vi "AG33XXX.ProcCases.vi"(0 "i ref in":refnum<vi>, 1 "selector":string, 2 "Data":T1, 3 "call cluster":T2={"Object"="", "Selector"="", "CallType"=enum."synchronous", "Async Object"="", "Async Selector"="", "Data Descriptor"="", "Data"=[], "Error #"=0, "Expire"=0}, 5 "error in (no error)":errorcluster) -> (14 "i ref out":refnum<vi>, 17 "answer cluster":T2={"Object"="", "Selector"="", "CallType"=enum."synchronous", "Async Object"="", "Async Selector"="", "Data Descriptor"="", "Data"=[], "Error #"=0, "Expire"=0}, 19 "error out":errorcluster)   [LabVIEW 2014, in "AG33XXX.lvlib"]
doc: "This method is called by a process from within the default case in the event loop. The methods of a class that are linked to events will be called from THIS method. Add your code here."
uses:
  AG33XXX.lvlib
  CSCore/CSSystem/CoreDefs/CoreDefs.call_type.ctl
  CSCore/BaseProcess/BaseProcess.descriptor string definition.ctl
  CSCore/CSSystem/CoreDefs/CoreDefs.rawDataType.ctl
  CSCore/CSSystem/CoreLib/CoreLib.string 2 byte array.vi
  CSCore/CSSystem/CoreLib/CoreLib.byte array 2 short.vi
  CSCore/CSSystem/CoreLib/CoreLib.byte array 2 string.vi
  CSCore/CSSystem/CoreLib/CoreLib.byte array 2 short array.vi
  CSCore/CSSystem/CoreLib/CoreLib.byte array 2 double.vi
  CSCore/CSSystem/CoreLib/CoreLib.lvlib
  CSCore/BaseProcess/BaseProcess.lvlib
  CSCore/CSApplicationBaseClasses/AFGBase/AFGBase.lvlib
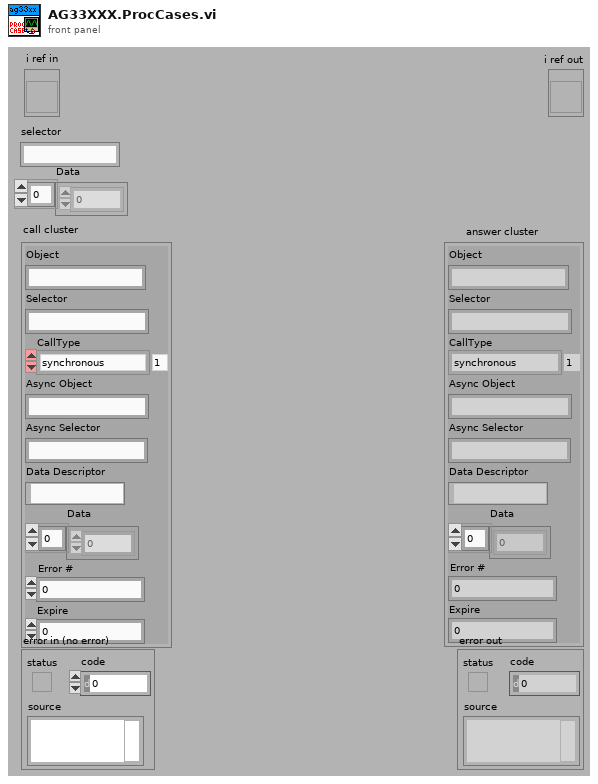
[diagram p1: front panel]
types:
  T1 = typedef "CoreDefs.rawDataType.ctl" = i8[]
  T2 = typedef "CoreDefs.call_type.ctl" = cluster{"Object":string, "Selector":string, "CallType":enum16{"simple", "synchronous", "asynchronous"}, "Async Object":string, "Async Selector":string, "Data Descriptor":T3, "Data":T1, "Error #":i32, "Expire":u32}
  T3 = typedef "BaseProcess.lvlib/BaseProcess.descriptor string definition.ctl" = string
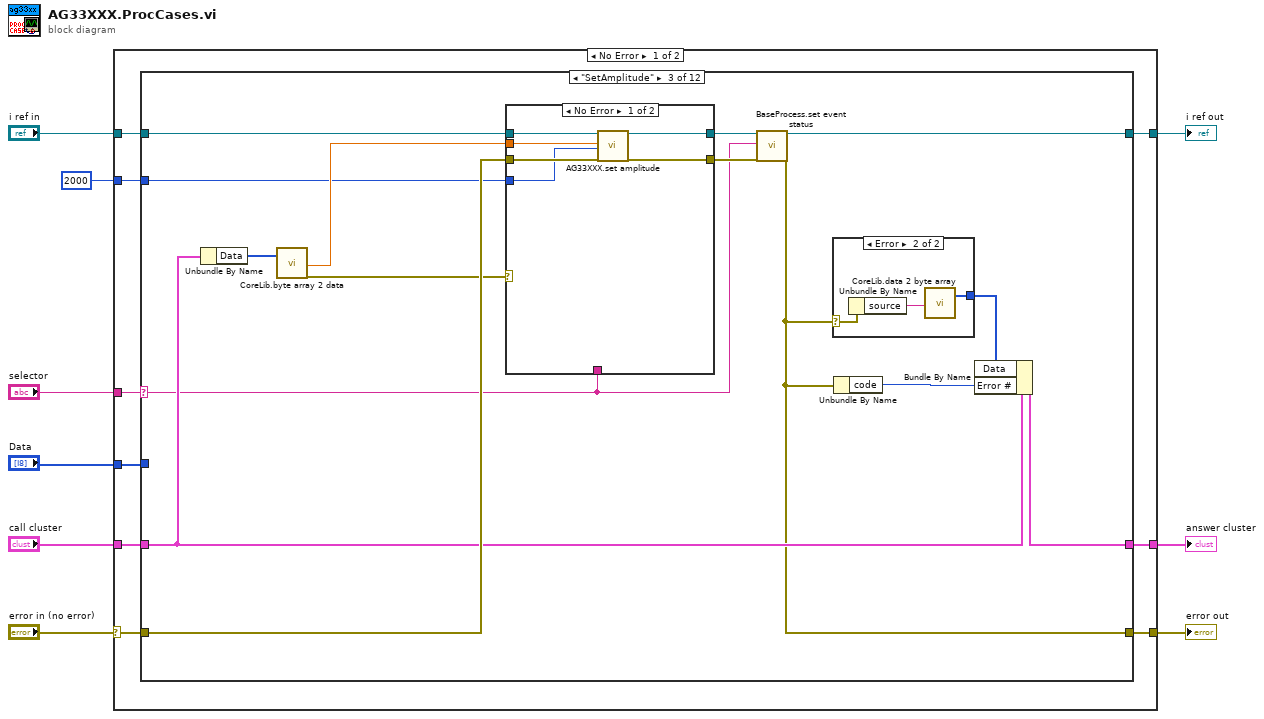
[diagram p0: block diagram]
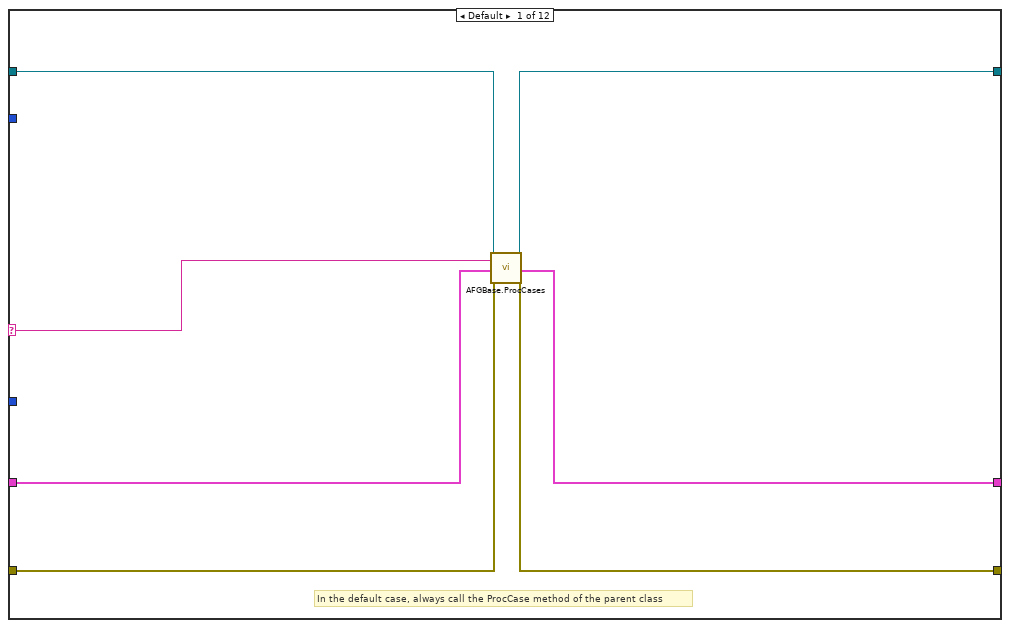
[diagram p2: hidden frame]
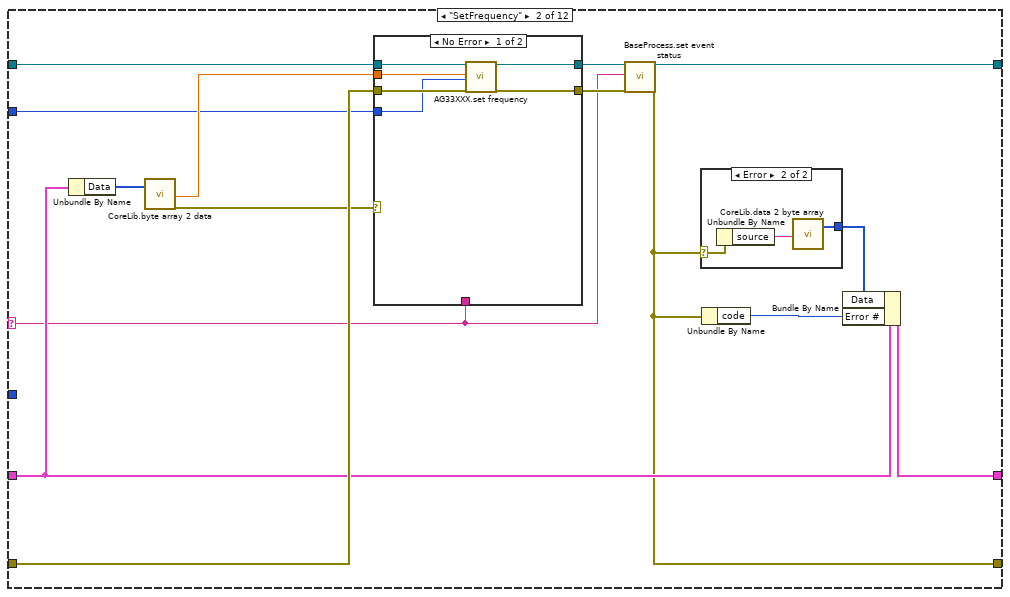
[diagram p3: hidden frame]
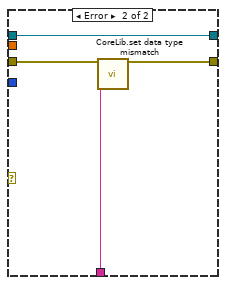
[diagram p5: hidden frame]
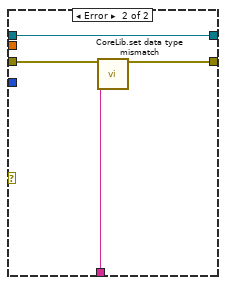
[diagram p7: hidden frame]
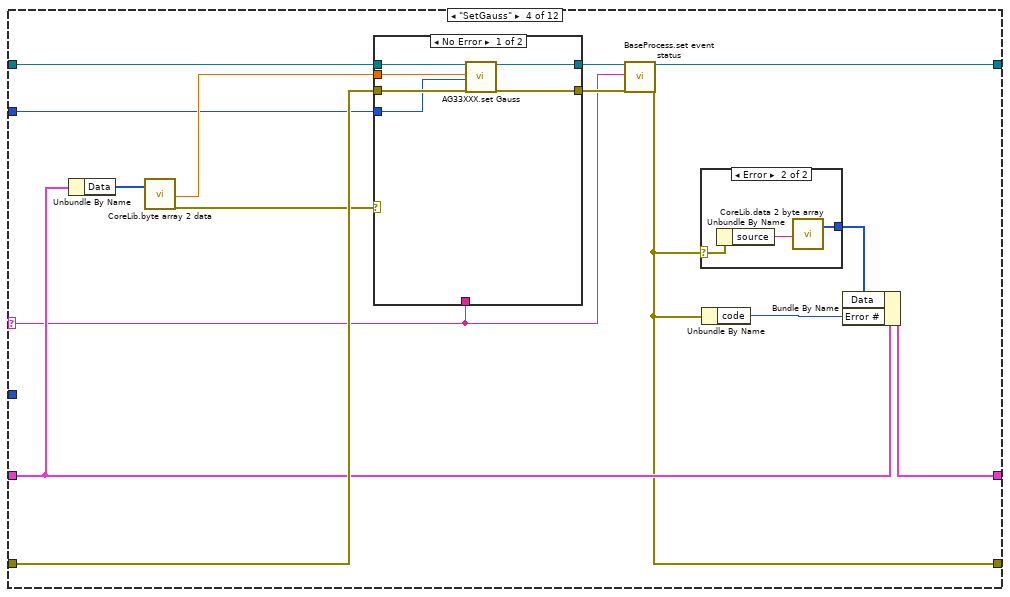
[diagram p8: hidden frame]
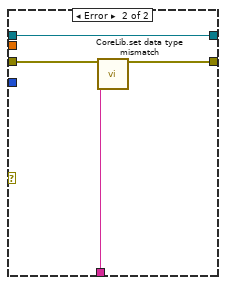
[diagram p10: hidden frame]
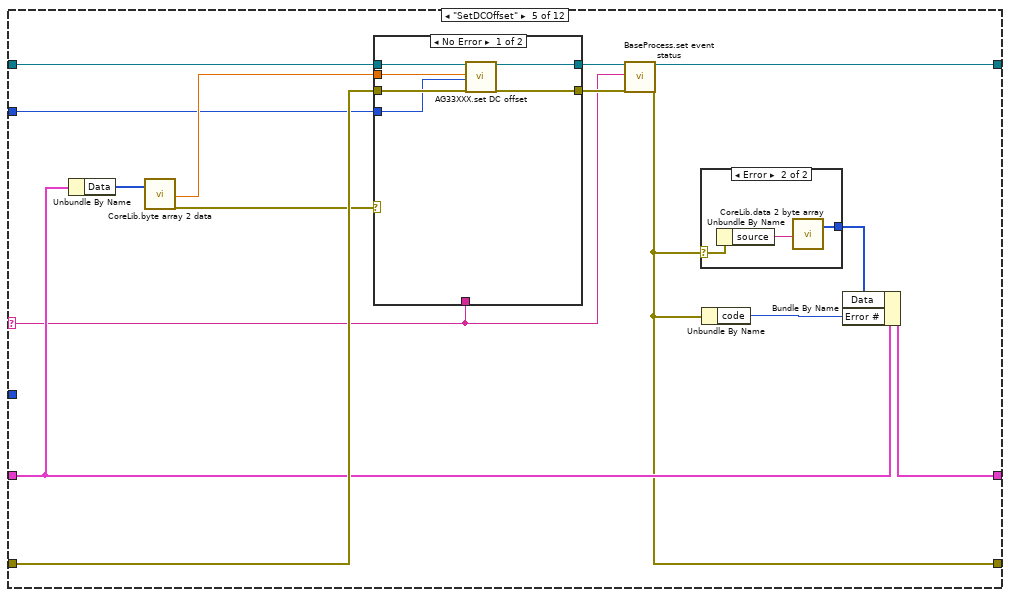
[diagram p11: hidden frame]
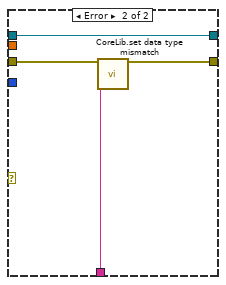
[diagram p13: hidden frame]
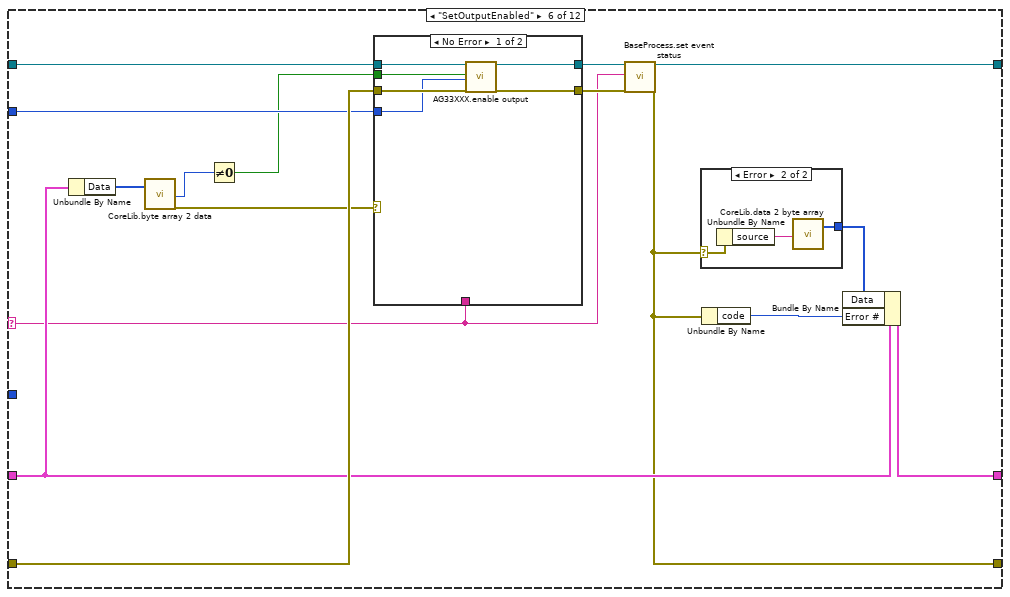
[diagram p14: hidden frame]
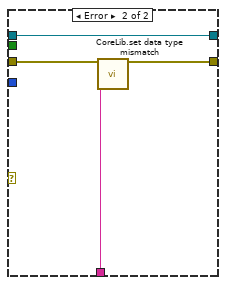
[diagram p16: hidden frame]
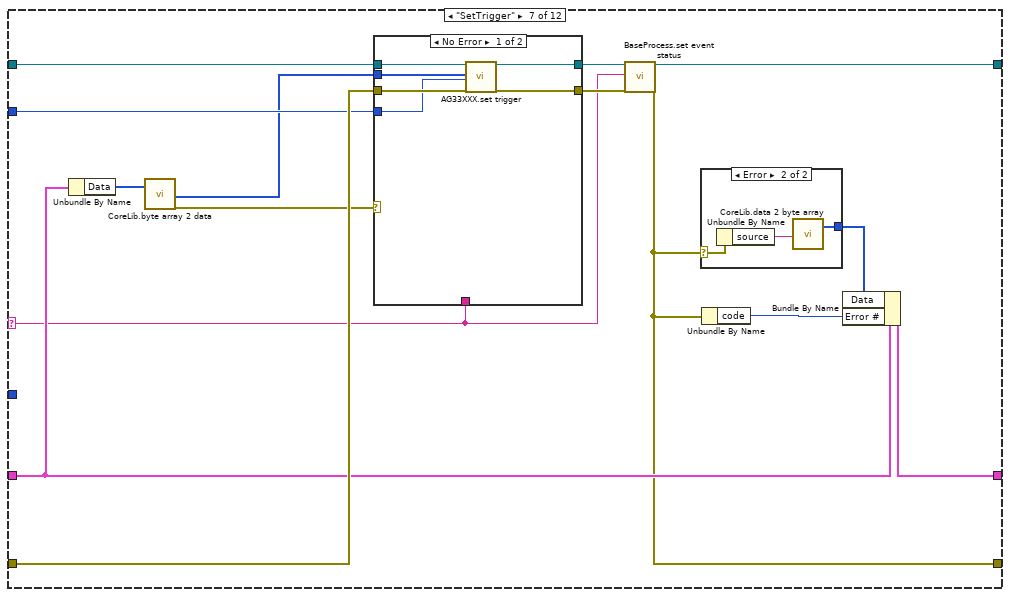
[diagram p17: hidden frame]
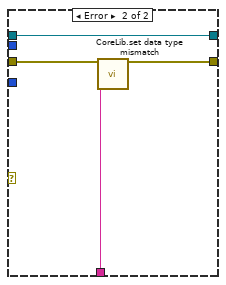
[diagram p19: hidden frame]
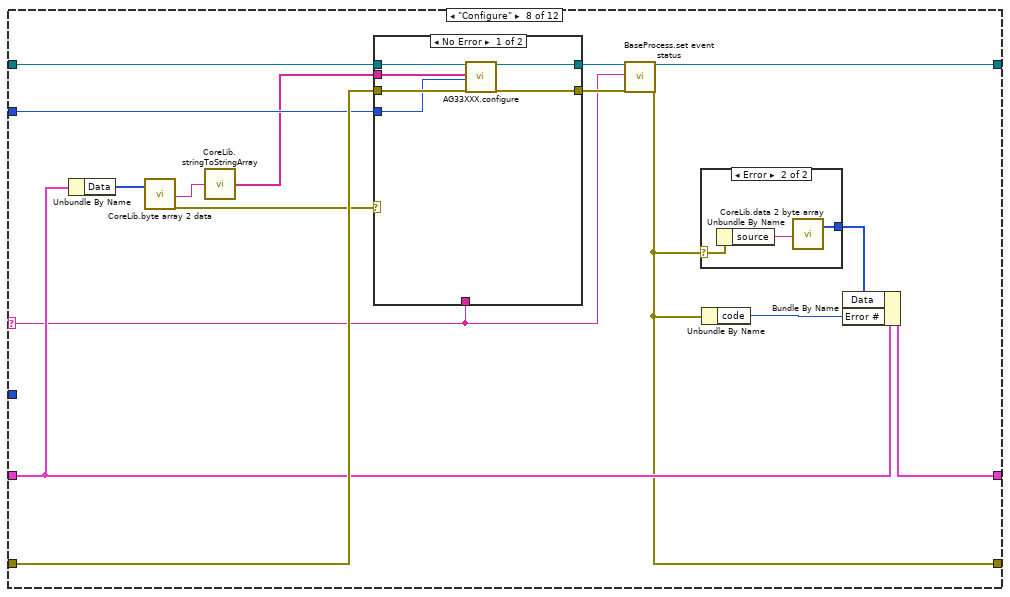
[diagram p20: hidden frame]
diagram:
  n1 = case shown="No Error" "error in (no error)" {
    selector: "error in (no error)" -> [w11 w310]
    tunnel: "selector" -> [w18 _]
    tunnel: [w17 w311] -> w8
    tunnel: "Data" -> [w16 _]
    tunnel: "call cluster" -> [w15 w311]
    tunnel: "i ref in" -> [w14 w312]
    tunnel: [w13 w312] -> w4
    tunnel: [w12 w310] -> w3
    tunnel: 2000 ("ms timeout (10000)") -> [w10 _]
    frame No Error {
      n2 = case shown="\"SetAmplitude\"" w18 {
        selector: w18 -> [w20 w31 w59 w87 w115 w144 w172 w201 w226 w241 w286 w301]
        tunnel: w16 -> [_ _ _ _ _ _ _ _ _ _ _ _]
        tunnel: w14 -> [w19 w40 w68 w96 w124 w153 w181 w210 w235 w249 w282 w297]
        tunnel: [w25 w30 w58 w86 w114 w143 w171 w200 w225 w252 w285 w300] -> w13
        tunnel: w15 -> [w21 w37 w65 w93 w121 w150 w178 w207 w232 w245 w290 w305]
        tunnel: [w22 w36 w64 w92 w120 w149 w177 w206 w231 w257 w289 w304] -> w17
        tunnel: w11 -> [w24 w39 w67 w95 w123 w152 w180 w209 w234 w250 w283 w298]
        tunnel: [w23 w32 w60 w88 w116 w145 w173 w202 w227 w253 w287 w302] -> w12
        tunnel: w10 -> [_ w26 w54 w82 w110 w139 w168 w197 w224 w251 w284 w299]
        frame Default {
          # "In the default case, always call the ProcCase method of the parent class"
          n3 = call "AFGBase.ProcCases.vi"("i ref in"=w19, "selector"=w20, "call cluster"=w21, "error in (no error)"=w24) -> ("i ref out"=w25:refnum<vi>, "answer cluster"=w22:T2, "error out"=w23:errorcluster)  [unwired: 13 in]
        }
        frame "SetFrequency" {
          n4 = Unbundle By Name(w37) -> ("Data"=w29:T1)
          n5 = call-poly "CoreLib.byte array 2 data.vi"("byteArray"=w29) -> ("d64"=w28:dbl, "error out"=w27:errorcluster)  [unwired: 16 in, 1 out]
          n6 = case shown="No Error" w27 {
            tunnel: [w48 w53] -> w34
            tunnel: w40 -> [w49 w53]
            tunnel: w39 -> [w46 w52]
            tunnel: [w47 w51] -> w33
            tunnel: w31 -> [_ w50]
            tunnel: w28 -> [w45 _]
            tunnel: w26 -> [w44 _]
            frame No Error {
              n7 = call "AG33XXX.set frequency.vi"("i ref in"=w49, "frequency [Hz]"=w45, "ms timeout (10000)"=w44, "error in (no error)"=w46) -> ("i ref out"=w48:refnum<vi>, "error out"=w47:errorcluster)  [unwired: 13 in, 1 out]
            }
            frame Error {
              n8 = call "CoreLib.set data type mismatch.vi"("error in (no error)"=w52, "error source"=w50) -> ("error out"=w51:errorcluster)  [unwired: 17 in]
            }
          }
          n9 = call "BaseProcess.set event status.vi"("i ref in"=w34, "EventStatus"=w31, "error in (no error)"=w33) -> ("i ref out"=w30:refnum<vi>, "error out"=w32:errorcluster)  [unwired: 14 in, 1 out]
          n10 = case shown="Error" w32 {
            selector: w32 -> [_ w43]
            tunnel: [_ w42] -> w35
            frame No Error {
            }
            frame Error {
              n11 = Unbundle By Name(w43) -> ("source"=w41:string)
              n12 = call-poly "CoreLib.data 2 byte array.vi"("string"=w41) -> ("byteArray out"=w42:T1)  [unwired: 18 in]
            }
          }
          n13 = Unbundle By Name(w32) -> ("code"=w38:i32)
          n14 = Bundle By Name(cluster=w37, "Data"=w35, "Error #"=w38) -> (w36:T2)
        }
        frame "SetAmplitude" {
          n15 = Unbundle By Name(w65) -> ("Data"=w57:T1)
          n16 = call-poly "CoreLib.byte array 2 data.vi"("byteArray"=w57) -> ("d64"=w56:dbl, "error out"=w55:errorcluster)  [unwired: 16 in, 1 out]
          n17 = case shown="No Error" w55 {
            tunnel: [w76 w81] -> w62
            tunnel: w68 -> [w77 w81]
            tunnel: w67 -> [w74 w80]
            tunnel: [w75 w79] -> w61
            tunnel: w59 -> [_ w78]
            tunnel: w56 -> [w73 _]
            tunnel: w54 -> [w72 _]
            frame No Error {
              n18 = call "AG33XXX.set amplitude.vi"("i ref in"=w77, "amplitude [V]"=w73, "ms timeout (10000)"=w72, "error in (no error)"=w74) -> ("i ref out"=w76:refnum<vi>, "error out"=w75:errorcluster)  [unwired: 13 in, 1 out]
            }
            frame Error {
              n19 = call "CoreLib.set data type mismatch.vi"("error in (no error)"=w80, "error source"=w78) -> ("error out"=w79:errorcluster)  [unwired: 17 in]
            }
          }
          n20 = call "BaseProcess.set event status.vi"("i ref in"=w62, "EventStatus"=w59, "error in (no error)"=w61) -> ("i ref out"=w58:refnum<vi>, "error out"=w60:errorcluster)  [unwired: 14 in, 1 out]
          n21 = case shown="Error" w60 {
            selector: w60 -> [_ w71]
            tunnel: [_ w70] -> w63
            frame No Error {
            }
            frame Error {
              n22 = Unbundle By Name(w71) -> ("source"=w69:string)
              n23 = call-poly "CoreLib.data 2 byte array.vi"("string"=w69) -> ("byteArray out"=w70:T1)  [unwired: 18 in]
            }
          }
          n24 = Unbundle By Name(w60) -> ("code"=w66:i32)
          n25 = Bundle By Name(cluster=w65, "Data"=w63, "Error #"=w66) -> (w64:T2)
        }
        frame "SetGauss" {
          n26 = Unbundle By Name(w93) -> ("Data"=w85:T1)
          n27 = call-poly "CoreLib.byte array 2 data.vi"("byteArray"=w85) -> ("d64"=w84:dbl, "error out"=w83:errorcluster)  [unwired: 16 in, 1 out]
          n28 = case shown="No Error" w83 {
            tunnel: [w104 w109] -> w90
            tunnel: w96 -> [w105 w109]
            tunnel: w95 -> [w102 w108]
            tunnel: [w103 w107] -> w89
            tunnel: w87 -> [_ w106]
            tunnel: w84 -> [w101 _]
            tunnel: w82 -> [w100 _]
            frame No Error {
              n29 = call "AG33XXX.set Gauss.vi"("i ref in"=w105, "Length [us]"=w101, "ms timeout (10000)"=w100, "error in (no error)"=w102) -> ("i ref out"=w104:refnum<vi>, "error out"=w103:errorcluster)  [unwired: 13 in, 1 out]
            }
            frame Error {
              n30 = call "CoreLib.set data type mismatch.vi"("error in (no error)"=w108, "error source"=w106) -> ("error out"=w107:errorcluster)  [unwired: 17 in]
            }
          }
          n31 = call "BaseProcess.set event status.vi"("i ref in"=w90, "EventStatus"=w87, "error in (no error)"=w89) -> ("i ref out"=w86:refnum<vi>, "error out"=w88:errorcluster)  [unwired: 14 in, 1 out]
          n32 = case shown="Error" w88 {
            selector: w88 -> [_ w99]
            tunnel: [_ w98] -> w91
            frame No Error {
            }
            frame Error {
              n33 = Unbundle By Name(w99) -> ("source"=w97:string)
              n34 = call-poly "CoreLib.data 2 byte array.vi"("string"=w97) -> ("byteArray out"=w98:T1)  [unwired: 18 in]
            }
          }
          n35 = Unbundle By Name(w88) -> ("code"=w94:i32)
          n36 = Bundle By Name(cluster=w93, "Data"=w91, "Error #"=w94) -> (w92:T2)
        }
        frame "SetDCOffset" {
          n37 = Unbundle By Name(w121) -> ("Data"=w113:T1)
          n38 = call-poly "CoreLib.byte array 2 data.vi"("byteArray"=w113) -> ("d64"=w112:dbl, "error out"=w111:errorcluster)  [unwired: 16 in, 1 out]
          n39 = case shown="No Error" w111 {
            tunnel: [w132 w137] -> w118
            tunnel: w124 -> [w133 w137]
            tunnel: w123 -> [w130 w136]
            tunnel: [w131 w135] -> w117
            tunnel: w115 -> [_ w134]
            tunnel: w112 -> [w129 _]
            tunnel: w110 -> [w128 _]
            frame No Error {
              n40 = call "AG33XXX.set DC offset.vi"("i ref in"=w133, "DCOffset [V]"=w129, "ms timeout (10000)"=w128, "error in (no error)"=w130) -> ("i ref out"=w132:refnum<vi>, "error out"=w131:errorcluster)  [unwired: 13 in, 1 out]
            }
            frame Error {
              n41 = call "CoreLib.set data type mismatch.vi"("error in (no error)"=w136, "error source"=w134) -> ("error out"=w135:errorcluster)  [unwired: 17 in]
            }
          }
          n42 = call "BaseProcess.set event status.vi"("i ref in"=w118, "EventStatus"=w115, "error in (no error)"=w117) -> ("i ref out"=w114:refnum<vi>, "error out"=w116:errorcluster)  [unwired: 14 in, 1 out]
          n43 = case shown="Error" w116 {
            selector: w116 -> [_ w127]
            tunnel: [_ w126] -> w119
            frame No Error {
            }
            frame Error {
              n44 = Unbundle By Name(w127) -> ("source"=w125:string)
              n45 = call-poly "CoreLib.data 2 byte array.vi"("string"=w125) -> ("byteArray out"=w126:T1)  [unwired: 18 in]
            }
          }
          n46 = Unbundle By Name(w116) -> ("code"=w122:i32)
          n47 = Bundle By Name(cluster=w121, "Data"=w119, "Error #"=w122) -> (w120:T2)
        }
        frame "SetOutputEnabled" {
          n48 = Unbundle By Name(w150) -> ("Data"=w142:T1)
          n49 = call-poly "CoreLib.byte array 2 data.vi"("byteArray"=w142) -> ("i16"=w141:i16, "error out"=w140:errorcluster)  [unwired: 16 in, 1 out]
          n50 = Not Equal To 0?(x=w141) -> (x != 0?=w138:bool)
          n51 = case shown="No Error" w140 {
            tunnel: [w161 w166] -> w147
            tunnel: w153 -> [w162 w166]
            tunnel: w152 -> [w159 w165]
            tunnel: [w160 w164] -> w146
            tunnel: w144 -> [_ w163]
            tunnel: w138 -> [w158 _]
            tunnel: w139 -> [w157 _]
            frame No Error {
              n52 = call "AG33XXX.enable output.vi"("i ref in"=w162, "outputEnable"=w158, "ms timeout (10000)"=w157, "error in (no error)"=w159) -> ("i ref out"=w161:refnum<vi>, "error out"=w160:errorcluster)  [unwired: 13 in, 1 out]
            }
            frame Error {
              n53 = call "CoreLib.set data type mismatch.vi"("error in (no error)"=w165, "error source"=w163) -> ("error out"=w164:errorcluster)  [unwired: 17 in]
            }
          }
          n54 = call "BaseProcess.set event status.vi"("i ref in"=w147, "EventStatus"=w144, "error in (no error)"=w146) -> ("i ref out"=w143:refnum<vi>, "error out"=w145:errorcluster)  [unwired: 14 in, 1 out]
          n55 = case shown="Error" w145 {
            selector: w145 -> [_ w156]
            tunnel: [_ w155] -> w148
            frame No Error {
            }
            frame Error {
              n56 = Unbundle By Name(w156) -> ("source"=w154:string)
              n57 = call-poly "CoreLib.data 2 byte array.vi"("string"=w154) -> ("byteArray out"=w155:T1)  [unwired: 18 in]
            }
          }
          n58 = Unbundle By Name(w145) -> ("code"=w151:i32)
          n59 = Bundle By Name(cluster=w150, "Data"=w148, "Error #"=w151) -> (w149:T2)
        }
        frame "SetTrigger" {
          n60 = Unbundle By Name(w178) -> ("Data"=w170:T1)
          n61 = call-poly "CoreLib.byte array 2 data.vi"("byteArray"=w170) -> ("[i16]"=w167:i16[], "error out"=w169:errorcluster)  [unwired: 16 in, 1 out]
          n62 = case shown="No Error" w169 {
            tunnel: [w189 w194] -> w175
            tunnel: w181 -> [w190 w194]
            tunnel: w180 -> [w187 w193]
            tunnel: [w188 w192] -> w174
            tunnel: w172 -> [_ w191]
            tunnel: w167 -> [w186 _]
            tunnel: w168 -> [w185 _]
            frame No Error {
              n63 = call "AG33XXX.set trigger.vi"("i ref in"=w190, "triggerParameters"=w186, "ms timeout (10000)"=w185, "error in (no error)"=w187) -> ("i ref out"=w189:refnum<vi>, "error out"=w188:errorcluster)  [unwired: 13 in, 1 out]
            }
            frame Error {
              n64 = call "CoreLib.set data type mismatch.vi"("error in (no error)"=w193, "error source"=w191) -> ("error out"=w192:errorcluster)  [unwired: 17 in]
            }
          }
          n65 = call "BaseProcess.set event status.vi"("i ref in"=w175, "EventStatus"=w172, "error in (no error)"=w174) -> ("i ref out"=w171:refnum<vi>, "error out"=w173:errorcluster)  [unwired: 14 in, 1 out]
          n66 = case shown="Error" w173 {
            selector: w173 -> [_ w184]
            tunnel: [_ w183] -> w176
            frame No Error {
            }
            frame Error {
              n67 = Unbundle By Name(w184) -> ("source"=w182:string)
              n68 = call-poly "CoreLib.data 2 byte array.vi"("string"=w182) -> ("byteArray out"=w183:T1)  [unwired: 18 in]
            }
          }
          n69 = Unbundle By Name(w173) -> ("code"=w179:i32)
          n70 = Bundle By Name(cluster=w178, "Data"=w176, "Error #"=w179) -> (w177:T2)
        }
        frame "Configure" {
          n71 = Unbundle By Name(w207) -> ("Data"=w199:T1)
          n72 = call-poly "CoreLib.byte array 2 data.vi"("byteArray"=w199) -> ("string"=w196:string, "error out"=w198:errorcluster)  [unwired: 16 in, 1 out]
          n73 = call "CoreLib.stringToStringArray.vi"("String"=w196) -> ("Array"=w195:string[])
          n74 = case shown="No Error" w198 {
            tunnel: [w218 w223] -> w204
            tunnel: w210 -> [w219 w223]
            tunnel: w209 -> [w216 w222]
            tunnel: [w217 w221] -> w203
            tunnel: w201 -> [_ w220]
            tunnel: w195 -> [w215 _]
            tunnel: w197 -> [w214 _]
            frame No Error {
              n75 = call "AG33XXX.configure.vi"("i ref in"=w219, "configureData"=w215, "ms timeout (10000)"=w214, "error in (no error)"=w216) -> ("i ref out"=w218:refnum<vi>, "error out"=w217:errorcluster)  [unwired: 13 in, 1 out]
            }
            frame Error {
              n76 = call "CoreLib.set data type mismatch.vi"("error in (no error)"=w222, "error source"=w220) -> ("error out"=w221:errorcluster)  [unwired: 17 in]
            }
          }
          n77 = call "BaseProcess.set event status.vi"("i ref in"=w204, "EventStatus"=w201, "error in (no error)"=w203) -> ("i ref out"=w200:refnum<vi>, "error out"=w202:errorcluster)  [unwired: 14 in, 1 out]
          n78 = case shown="Error" w202 {
            selector: w202 -> [_ w213]
            tunnel: [_ w212] -> w205
            frame No Error {
            }
            frame Error {
              n79 = Unbundle By Name(w213) -> ("source"=w211:string)
              n80 = call-poly "CoreLib.data 2 byte array.vi"("string"=w211) -> ("byteArray out"=w212:T1)  [unwired: 18 in]
            }
          }
          n81 = Unbundle By Name(w202) -> ("code"=w208:i32)
          n82 = Bundle By Name(cluster=w207, "Data"=w205, "Error #"=w208) -> (w206:T2)
        }
        frame "UseAM" {
          n83 = call "AG33XXX.use external amplitude modulation.vi"("i ref in"=w235, "ms timeout (10000)"=w224, "error in (no error)"=w234) -> ("i ref out"=w229:refnum<vi>, "error out"=w228:errorcluster)  [unwired: 14 in, 1 out]
          n84 = call "BaseProcess.set event status.vi"("i ref in"=w229, "EventStatus"=w226, "error in (no error)"=w228) -> ("i ref out"=w225:refnum<vi>, "error out"=w227:errorcluster)  [unwired: 14 in, 1 out]
          n85 = case shown="Error" w227 {
            selector: w227 -> [_ w238]
            tunnel: [_ w237] -> w230
            frame No Error {
            }
            frame Error {
              n86 = Unbundle By Name(w238) -> ("source"=w236:string)
              n87 = call-poly "CoreLib.data 2 byte array.vi"("string"=w236) -> ("byteArray out"=w237:T1)  [unwired: 18 in]
            }
          }
          n88 = Unbundle By Name(w227) -> ("code"=w233:i32)
          n89 = Bundle By Name(cluster=w232, "Data"=w230, "Error #"=w233) -> (w231:T2)
        }
        frame "Initialize" {
          n90 = Unbundle By Name(w245) -> ("Data"=w246:T1)
          n91 = call-poly "CoreLib.byte array 2 data.vi"("byteArray"=w246) -> ("byteArray out"=w244:T1, "i16"=w240:i16, "error out"=w243:errorcluster)  [unwired: 16 in]
          n92 = call-poly "CoreLib.byte array 2 data.vi"("byteArray"=w244, "error in (no error)"=w243) -> ("i16"=w239:i16, "error out"=w242:errorcluster)  [unwired: 15 in, 1 out]
          n93 = case shown="No Error" w242 {
            tunnel: [w270 w274] -> w255
            tunnel: [w269 w272] -> w254
            tunnel: w251 -> [w268 _]
            tunnel: w250 -> [w266 w273]
            tunnel: w249 -> [w265 w274]
            tunnel: [w263 _] -> w248
            tunnel: w241 -> [_ w271]
            tunnel: w240 -> [w262 _]
            tunnel: w239 -> [w260 _]
            frame No Error {
              n94 = Not Equal To 0?(x=w262) -> (x != 0?=w261:bool)
              n95 = Not Equal To 0?(x=w260) -> (x != 0?=w259:bool)
              n96 = call "AG33XXX.close.vi"("i ref in"=w265, "ms timeout (10000)"=w268, "error in (no error)"=w266) -> ("i ref out"=w264:refnum<vi>, "error out"=w267:errorcluster)  [unwired: 14 in, 1 out]
              n97 = call "AG33XXX.initialize.vi"("i ref in"=w264, "queryID"=w261, "resetDevice"=w259, "ms timeout (10000)"=w268, "error in (no error)"=w267) -> ("i ref out"=w270:refnum<vi>, "deviceID"=w263:string, "error out"=w269:errorcluster)  [unwired: 11 in, 1 out]
            }
            frame Error {
              n98 = call "CoreLib.set data type mismatch.vi"("error in (no error)"=w273, "error source"=w271) -> ("error out"=w272:errorcluster)  [unwired: 17 in]
            }
          }
          n99 = call "BaseProcess.set event status.vi"("i ref in"=w255, "EventStatus"=w241, "error in (no error)"=w254) -> ("i ref out"=w252:refnum<vi>, "error out"=w253:errorcluster)  [unwired: 14 in, 1 out]
          n100 = case shown="No Error" w253 {
            selector: w253 -> [_ w279]
            tunnel: [w276 w278] -> w256
            tunnel: w248 -> [w275 _]
            frame No Error {
              n101 = call-poly "CoreLib.data 2 byte array.vi"("string"=w275) -> ("byteArray out"=w276:T1)  [unwired: 18 in]
            }
            frame Error {
              n102 = Unbundle By Name(w279) -> ("source"=w277:string)
              n103 = call-poly "CoreLib.data 2 byte array.vi"("string"=w277) -> ("byteArray out"=w278:T1)  [unwired: 18 in]
            }
          }
          n104 = Unbundle By Name(w253) -> ("code"=w258:i32)
          n105 = Bundle By Name(cluster=w245, "Data"=w256, "Error #"=w258, "Data Descriptor"=T3 "C:N") -> (w257:T2)
        }
        frame "Close" {
          n106 = call "AG33XXX.close.vi"("i ref in"=w282, "ms timeout (10000)"=w284, "error in (no error)"=w283) -> ("i ref out"=w281:refnum<vi>, "error out"=w280:errorcluster)  [unwired: 14 in, 1 out]
          n107 = call "BaseProcess.set event status.vi"("i ref in"=w281, "EventStatus"=w286, "error in (no error)"=w280) -> ("i ref out"=w285:refnum<vi>, "error out"=w287:errorcluster)  [unwired: 14 in, 1 out]
          n108 = case shown="Error" w287 {
            selector: w287 -> [_ w294]
            tunnel: [_ w293] -> w288
            frame No Error {
            }
            frame Error {
              n109 = Unbundle By Name(w294) -> ("source"=w292:string)
              n110 = call-poly "CoreLib.data 2 byte array.vi"("string"=w292) -> ("byteArray out"=w293:T1)  [unwired: 18 in]
            }
          }
          n111 = Unbundle By Name(w287) -> ("code"=w291:i32)
          n112 = Bundle By Name(cluster=w290, "Data"=w288, "Error #"=w291) -> (w289:T2)
        }
        frame "Reset" {
          n113 = call "AG33XXX.reset.vi"("i ref in"=w297, "ms timeout (10000)"=w299, "error in (no error)"=w298) -> ("i ref out"=w296:refnum<vi>, "error out"=w295:errorcluster)  [unwired: 14 in, 1 out]
          n114 = call "BaseProcess.set event status.vi"("i ref in"=w296, "EventStatus"=w301, "error in (no error)"=w295) -> ("i ref out"=w300:refnum<vi>, "error out"=w302:errorcluster)  [unwired: 14 in, 1 out]
          n115 = case shown="Error" w302 {
            selector: w302 -> [_ w309]
            tunnel: [_ w308] -> w303
            frame No Error {
            }
            frame Error {
              n116 = Unbundle By Name(w309) -> ("source"=w307:string)
              n117 = call-poly "CoreLib.data 2 byte array.vi"("string"=w307) -> ("byteArray out"=w308:T1)  [unwired: 18 in]
            }
          }
          n118 = Unbundle By Name(w302) -> ("code"=w306:i32)
          n119 = Bundle By Name(cluster=w305, "Data"=w303, "Error #"=w306) -> (w304:T2)
        }
      }
    }
    frame Error {
    }
  }
  "answer cluster" <- w8
  "i ref out" <- w4
  "error out" <- w3
